vi "MT Generate Symbol Map (Circular).vi"(0 "symbol values":i32[][](array[numeric]), 5 "symbol phases (degrees)":dbl[][](array[numeric]), 7 "symbol radii":dbl[](array[numeric]), 11 "error in (no error)":errorcluster) -> (4 "symbol map":cdb[](array[numeric]) format="%.3f", 15 "error out":errorcluster)   [LabVIEW 2020, in "niDMT.lvlib"]
doc: "This polymorphic instance generates a symbol map, using the matrix of <B>symbol values</B> that you specify, a matrix representing the symbol phases in degrees, and an array representing the radii of each discrete circle. Use the <B>symbol map</B> parameter of the <B>system parameters</B> cluster to configure the operation of the demodulation and modulation VIs.\n\nThe <B>symbol values</B> matrix defines how the M-ary binary data are mapped to the discrete I/Q symbols on the constellation diagram. The VI maps the specified symbol values to I/Q constellation points using the polar representation . The VI reads the <B>symbol values/symbol phases</B> matrices row-wise. Each row of symbol values/symbol phases is then mapped onto I/Q symbol points, which are located on a circle with a radius that is specified in the <B>symbol radii</B> array.\n\n<B>NOTE:</B> The dimensions of the symbol amplitudes matrix must exactly match the dimensions of the"
uses:
  <vilib>/addons/Modulation/niDMT.lvlib
  <vilib>/addons/Modulation/niAMT.lvlib
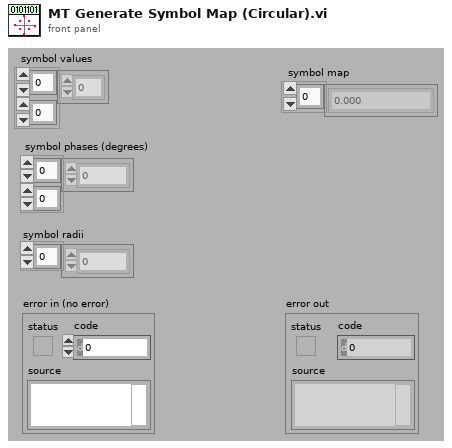
[diagram p1: front panel]
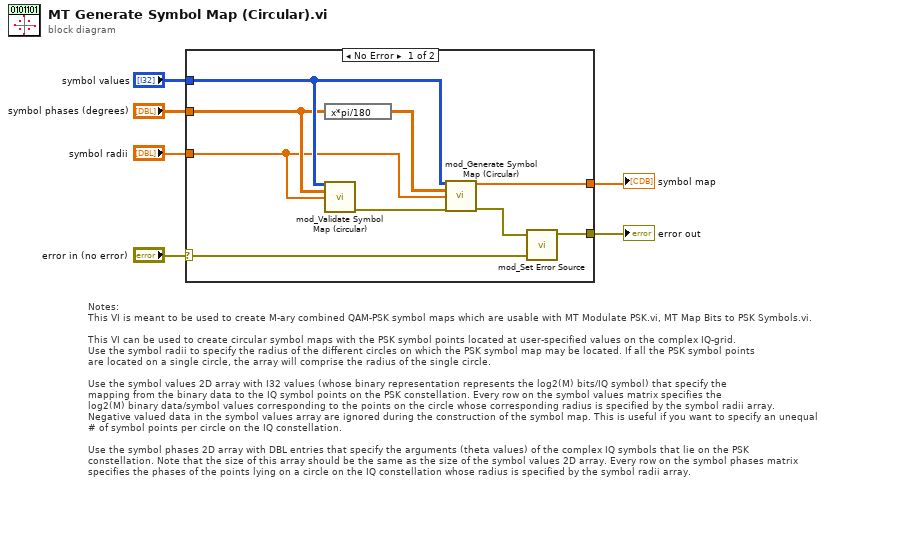
[diagram p0: block diagram]
diagram:
  # "Notes:\nThis VI is meant to be used to create M-ary combined QAM-PSK symbol maps which are usable with MT Modulate PSK.vi, MT Map Bits to PSK Symbols.vi.\n\nThis VI can be used to create circular symbol maps with the PSK symbol points located at user-specified values on the complex IQ-grid.\nUse the symbol radii to specify the radius of the different circles on which the PSK symbol map may be located. If all the PSK symbol points\nare located on a single circle, the array will comprise the radius of the single circle.\n\nUse the symbol values 2D array with I32 values (whose binary representation represents the log2(M) bits/IQ symbol) that specify the \nmapping from the binary data to the IQ symbol points on the PSK constellation. Every row on the symbol values matrix specifies the \nlog2(M) binary data/symbol values corresponding to the points on the circle whose corresponding radius is specified by the symbol radii array. \nNegative valued data in the symbol values array are ignored during the construction of the symbol map. This is useful if you want to specify an unequal\n# of symbol points per circle on the IQ constellation.\n\nUse the symbol phases 2D array with DBL entries that specify the arguments (theta values) of the complex IQ symbols that lie on the PSK \nconstellation. Note that the size of this array should be the same as the size of the symbol values 2D array. Every row on the symbol phases matrix\nspecifies the phases of the points lying on a circle on the IQ constellation whose radius is specified by the symbol radii array."
  n1 = case shown="No Error" "error in (no error)" {
    selector: "error in (no error)" -> [w11 _]
    tunnel: "symbol values" -> [w9 _]
    tunnel: [w15 _] -> w5
    tunnel: [w12 _] -> w3
    tunnel: "symbol radii" -> [w7 _]
    tunnel: "symbol phases (degrees)" -> [w8 _]
    frame No Error {
      n2 = expression code="x*pi/180"(w8) -> (w14:dbl[][])
      n3 = call <vilib>:"mod_Validate Symbol Map (circular).vi"("symbol values"=w9, "symbol phases (degrees)"=w8, "symbol radii"=w7) -> ("error out"=w10:errorcluster)  [unwired: 12 out]
      n4 = call <vilib>:"mod_Generate Symbol Map (Circular).vi"("symbol values"=w9, "symbol phases\n(radians)"=w14, "symbol radii"=w7, "error in (no error)"=w10) -> ("symbol map"=w15:cdb[], "error out"=w13:errorcluster)  [unwired: 10 out]
      n5 = call <vilib>:"mod_Set Error Source.vi"("initial error in (no error)"=w11, "final error in (no error)"=w13) -> ("error out"=w12:errorcluster)  [unwired: 3 out]
    }
    frame Error {
    }
  }
  "symbol map" <- w5
  "error out" <- w3
